vi "Move to Inst Pos.vi"(8 "error in (no error)":errorcluster, 10 "Inst Pos":i32, 11 "FujiMotor in":refnum<class "FujiMotor.lvclass">) -> (0 "error out":errorcluster, 3 "FujiMotor out":refnum<class "FujiMotor.lvclass">)   [LabVIEW 2014, in "ALPHA5 RS485.lvlib" / "FujiMotor.lvclass"]
uses:
  FujiMotor.lvclass
  FujiMotor.lvclass/FujiMotor.ctl
  ALPHA5 RS485.lvlib
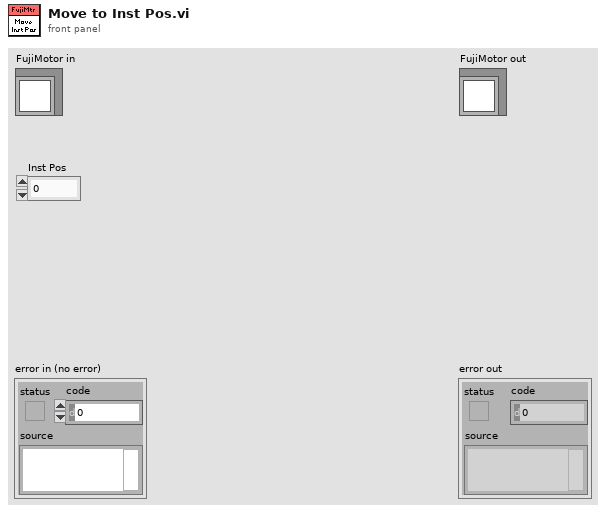
[diagram p1: front panel]
types:
  T1 = typedef "ALPHA5 RS485.lvlib/Port Selection Info.ctl" = cluster{"Port Name":refnum<visa-resource-name>, "Amplifier Num":u8, "Baud Rate":u32, "Char Formation":enum16{"0", "1", "2", "3", "4", "5"}}
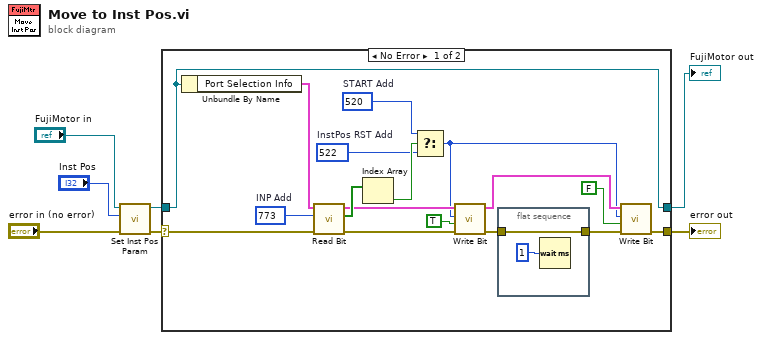
[diagram p0: block diagram]
diagram:
  n1 = call "Set Inst Pos Param.vi"("error in (no error)"="error in (no error)", "Inst Pos"="Inst Pos", "FujiMotor in"="FujiMotor in") -> ("error out"=w1:errorcluster, "FujiMotor out"=w3:refnum<class "FujiMotor.lvclass">)  [unwired: 7 in]
  n2 = case shown="No Error" w1 {
    selector: w1 -> [w22 w27]
    tunnel: [w8 w27] -> w7
    tunnel: [w24 w28] -> w6
    tunnel: w3 -> [w24 w28]
    frame No Error {
      w17 = u16 522  # InstPos RST Add
      w18 = u16 520  # START Add
      w21 = u16 773  # INP Add
      n3 = Unbundle By Name(w24) -> ("Port Selection Info"=w23:T1)
      n4 = call "Read Bit.vi"("error in (no error)"=w22, "Address"=w21, "Port Selection Info In"=w23) -> ("error out"=w15:errorcluster, "bits array"=w20:bool[], "Port Selection Info Out"=w16:T1)  [unwired: 6 in]
      n5 = Index Array(array=w20) -> (element=w19:bool)  [unwired: 1 in]
      n6 = Select(t=w18, s=w19, f=w17) -> (s? t:f=w10:u16)
      n7 = call "Write Bit.vi"("error in (no error)"=w15, "ON/OFF"=TRUE, "Address"=w10, "Port Selection Info In"=w16) -> ("error out"=w13:errorcluster, "Port Selection Info Out"=w11:T1)  [unwired: 6 in]
      n8 = flat-sequence {
        tunnel: w13 -> [w25]
        tunnel: [w25] -> w12
        frame #0 {
          n9 = Wait (ms)(milliseconds to wait=u32 1) -> ()  [unwired: 1 out]
        }
      }
      n10 = call "Write Bit.vi"("error in (no error)"=w12, "ON/OFF"=FALSE, "Address"=w10, "Port Selection Info In"=w11) -> ("error out"=w8:errorcluster)  [unwired: 6 in, 1 out]
    }
    frame Error {
    }
  }
  "error out" <- w7
  "FujiMotor out" <- w6
